vi "SCPI_GET_REFOSC_SRC.vi"(8 "error in":errorcluster {"code" format="%.0x"}, 11 "Session In":refnum<visa-resource-name>="GPIB0::16::INSTR") -> (0 "error out":errorcluster {"code" format="%.0x"}, 2 "REF OSC SOURCE":string, 3 "Session Out":refnum<visa-resource-name>)   [LabVIEW 2018]
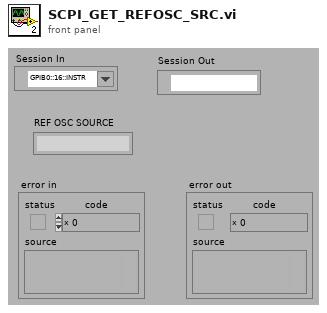
[diagram p1: front panel]
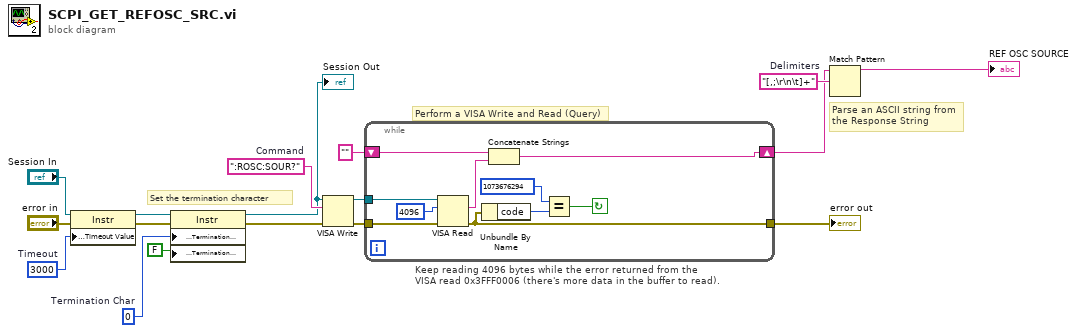
[diagram p0: block diagram]
diagram:
  w3 = "[,;\r\n\t]+"  # Delimiters
  w5 = ":ROSC:SOUR?"  # Command
  w12 = u8 0  # Termination Char
  w17 = u32 3000  # Timeout
  # "Parse an ASCII string from the Response String"
  # "Perform a VISA Write and Read (Query)"
  # "Keep reading 4096 bytes while the error returned from the\nVISA read 0x3FFF0006 (there's more data in the buffer to read)."
  # "Set the termination character"
  n1 = property class="Instr"(reference="Session In", error in="error in", "General Settings:Timeout Value"=w17) -> (reference out=w11:refnum<visa-resource-name>, error out=w14:errorcluster)
  n2 = property class="Instr"(reference=w11, error in=w14, "Message Based Settings:Termination Character"=w12, "Message Based Settings:Termination Character Enable"=FALSE ("enable")) -> (reference out=w1:refnum<visa-resource-name>, error out=w13:errorcluster)
  "Session Out" <- w1
  n3 = VISA Write(VISA resource name=w1, write buffer=w5, error in (no error)=w13) -> (VISA resource name out=w9:refnum<visa-resource-name>, error out=w8:errorcluster)  [unwired: 1 out]
  n4 = while {
    tunnel: w9 -> [w24]
    shift-right: [w18] -> w2
    shift-left: "" -> [w23]
    tunnel: w8 -> [w21]
    tunnel: [w20] -> w7
    stop <- w19 continue-if-true
    n5 = VISA Read(VISA resource name=w24, byte count=u32 4096 ("byte count (0)"), error in (no error)=w21) -> (read buffer=w22:string, error out=w20:errorcluster)  [unwired: 2 out]
    n6 = Unbundle By Name(w20) -> ("code"=w26:i32)
    n7 = Concatenate Strings(w23, w22) -> (w18:string)
    n8 = Equal?(x=1073676294, y=w26) -> (x = y?=w19:bool)
  }
  "error out" <- w7
  n9 = Match Pattern(string=w2, regular expression=w3) -> (before substring=→"REF OSC SOURCE":string)  [unwired: 4 out]
